vi "WLAN - niVST - RFSG - Create and Down Load Wfm.vi"(0 "instrument handle":refnum<k15>, 1 "Waveform Generation Settings":T2[](array[typedef])=[{"Standard"=0, "Channel Bandwidth (Hz)"=20000000.0, "Idle Interval (s)"=0.0001, "MCS Index"=0, "80211n PLCP Frame Format"=0, "Payload Data Length (bytes)"=100, "OFDM Data Rate (Mbps)"=0, "DSSS Data Rate (Mbps)"=0, "Wfm_Index"=0}, {"Standard"=0, "Channel Bandwidth (Hz)"=20000000.0, "Idle Interval (s)"=0.001, "MCS Index"=0, "80211n PLCP Frame Format"=0, "Payload Data Length (bytes)"=200, "OFDM Data Rate (Mbps)"=2, "DSSS Data Rate (Mbps)"=0, "Wfm_Index"=1}, {"Standard"=0, "Channel Bandwidth (Hz)"=20000000.0, "Idle Interval (s)"=0.0001, "MCS Index"=0, "80211n PLCP Frame Format"=0, "Payload Data Length (bytes)"=300, "OFDM Data Rate (Mbps)"=4, "DSSS Data Rate (Mbps)"=0, "Wfm_Index"=2}, {"Standard"=0, "Channel Bandwidth (Hz)"=20000000.0, "Idle Interval (s)"=0.0001, "MCS Index"=0, "80211n PLCP Frame Format"=0, "Payload Data Length (bytes)"=600, "OFDM Data Rate (Mbps)"=7, "DSSS Data Rate (Mbps)"=0, "Wfm_Index"=3}, {"Standard"=1, "Channel Bandwidth (Hz)"=20000000.0, "Idle Interval (s)"=0.0001, "MCS Index"=0, "80211n PLCP Frame Format"=0, "Payload Data Length (bytes)"=50, "OFDM Data Rate (Mbps)"=0, "DSSS Data Rate (Mbps)"=0, "Wfm_Index"=4}, {"Standard"=1, "Channel Bandwidth (Hz)"=20000000.0, "Idle Interval (s)"=0.0001, "MCS Index"=0, "80211n PLCP Frame Format"=0, "Payload Data Length (bytes)"=200, "OFDM Data Rate (Mbps)"=0, "DSSS Data Rate (Mbps)"=4, "Wfm_Index"=5}, {"Standard"=3, "Channel Bandwidth (Hz)"=20000000.0, "Idle Interval (s)"=0.0001, "MCS Index"=0, "80211n PLCP Frame Format"=0, "Payload Data Length (bytes)"=80, "OFDM Data Rate (Mbps)"=0, "DSSS Data Rate (Mbps)"=0, "Wfm_Index"=6}, {"Standard"=3, "Channel Bandwidth (Hz)"=20000000.0, "Idle Interval (s)"=0.0001, "MCS Index"=4, "80211n PLCP Frame Format"=0, "Payload Data Length (bytes)"=200, "OFDM Data Rate (Mbps)"=0, "DSSS Data Rate (Mbps)"=0, "Wfm_Index"=7}, {"Standard"=3, "Channel Bandwidth (Hz)"=20000000.0, "Idle Interval (s)"=0.0001, "MCS Index"=7, "80211n PLCP Frame Format"=0, "Payload Data Length (bytes)"=700, "OFDM Data Rate (Mbps)"=0, "DSSS Data Rate (Mbps)"=0, "Wfm_Index"=8}, {"Standard"=0, "Channel Bandwidth (Hz)"=20000000.0, "Idle Interval (s)"=0.0001, "MCS Index"=0, "80211n PLCP Frame Format"=0, "Payload Data Length (bytes)"=60, "OFDM Data Rate (Mbps)"=0, "DSSS Data Rate (Mbps)"=0, "Wfm_Index"=9}, {"Standard"=0, "Channel Bandwidth (Hz)"=20000000.0, "Idle Interval (s)"=0.0001, "MCS Index"=0, "80211n PLCP Frame Format"=0, "Payload Data Length (bytes)"=200, "OFDM Data Rate (Mbps)"=2, "DSSS Data Rate (Mbps)"=0, "Wfm_Index"=10}, {"Standard"=0, "Channel Bandwidth (Hz)"=20000000.0, "Idle Interval (s)"=0.0001, "MCS Index"=0, "80211n PLCP Frame Format"=0, "Payload Data Length (bytes)"=300, "OFDM Data Rate (Mbps)"=4, "DSSS Data Rate (Mbps)"=0, "Wfm_Index"=11}, {"Standard"=0, "Channel Bandwidth (Hz)"=20000000.0, "Idle Interval (s)"=0.0001, "MCS Index"=0, "80211n PLCP Frame Format"=0, "Payload Data Length (bytes)"=600, "OFDM Data Rate (Mbps)"=7, "DSSS Data Rate (Mbps)"=0, "Wfm_Index"=12}, {"Standard"=3, "Channel Bandwidth (Hz)"=20000000.0, "Idle Interval (s)"=0.0001, "MCS Index"=0, "80211n PLCP Frame Format"=0, "Payload Data Length (bytes)"=80, "OFDM Data Rate (Mbps)"=0, "DSSS Data Rate (Mbps)"=0, "Wfm_Index"=13}, {"Standard"=3, "Channel Bandwidth (Hz)"=20000000.0, "Idle Interval (s)"=0.0001, "MCS Index"=4, "80211n PLCP Frame Format"=0, "Payload Data Length (bytes)"=300, "OFDM Data Rate (Mbps)"=0, "DSSS Data Rate (Mbps)"=0, "Wfm_Index"=14}, {"Standard"=3, "Channel Bandwidth (Hz)"=20000000.0, "Idle Interval (s)"=0.0001, "MCS Index"=7, "80211n PLCP Frame Format"=0, "Payload Data Length (bytes)"=600, "OFDM Data Rate (Mbps)"=0, "DSSS Data Rate (Mbps)"=0, "Wfm_Index"=15}, {"Standard"=3, "Channel Bandwidth (Hz)"=40000000.0, "Idle Interval (s)"=0.0001, "MCS Index"=0, "80211n PLCP Frame Format"=0, "Payload Data Length (bytes)"=120, "OFDM Data Rate (Mbps)"=0, "DSSS Data Rate (Mbps)"=0, "Wfm_Index"=16}, {"Standard"=3, "Channel Bandwidth (Hz)"=40000000.0, "Idle Interval (s)"=0.0001, "MCS Index"=4, "80211n PLCP Frame Format"=0, "Payload Data Length (bytes)"=400, "OFDM Data Rate (Mbps)"=0, "DSSS Data Rate (Mbps)"=0, "Wfm_Index"=17}, {"Standard"=3, "Channel Bandwidth (Hz)"=40000000.0, "Idle Interval (s)"=0.0001, "MCS Index"=7, "80211n PLCP Frame Format"=0, "Payload Data Length (bytes)"=1024, "OFDM Data Rate (Mbps)"=0, "DSSS Data Rate (Mbps)"=0, "Wfm_Index"=18}] {"DSSS Data Rate (Mbps)" items=["1", "2", "5.5 CCK", "5.5 PBCC", "11 CCK", "11 PBCC", "22", "33"]; "OFDM Data Rate (Mbps)" items=["6", "9", "12", "18", "24", "36", "48", "54"]; "80211n PLCP Frame Format" items=["Mixed Format", "Greenfield Format"]; "Standard" items=["80211A/G/J/P OFDM", "80211B/G DSSS", "80211G DSSSOFDM", "80211N MIMOOFDM", "80211AC MIMOOFDM"]}, 2 "ScriptName<index>":string="WLANRxTesting", 11 "error in":errorcluster, 12 "Address String":string="00:90:4C:C5:12:38", 13 "numPackets":i32=100) -> (4 "instrument handle":refnum<k15>, 6 "Test Paramaters":T1[](array[typedef]) {"OFDM Data Rate (Mbps)" items=["6", "9", "12", "18", "24", "36", "48", "54"]; "DSSS Data Rate (Mbps)" items=["1", "2", "5.5 CCK", "5.5 PBCC", "11 CCK", "11 PBCC", "22", "33"]; "80211n PLCP Frame Format" items=["Mixed Format", "Greenfield Format"]}, 15 "error out":errorcluster)   [LabVIEW 2011]
uses:
  TV/RW/Includes/WLAN - TV - RW - INC - Rx_PER_Wfm_Settings.ctl
  TV/RW/Includes/WLAN - TV - RW - INC - RxTestParameters.ctl
  <instrlib>/niRFSG/niRFSG.llb/niRFSG Write Arb Waveform (Complex Input).vi
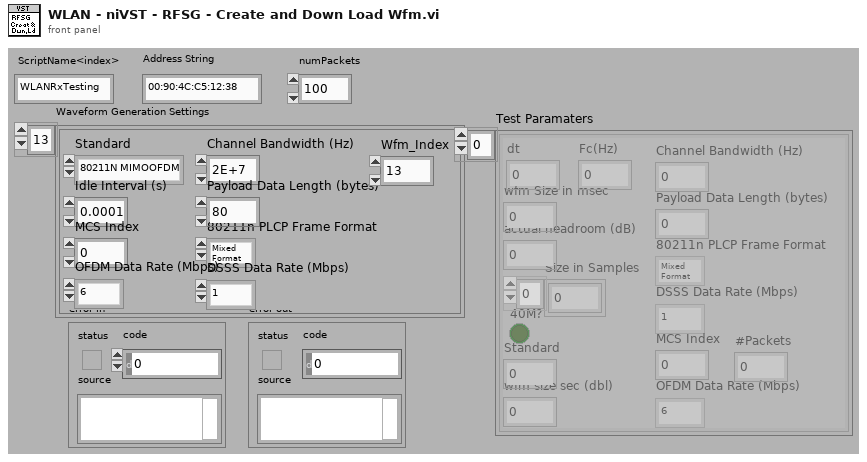
[diagram p1: front panel]
types:
  T1 = typedef "WLAN - TV - RW - INC - RxTestParameters.ctl" = cluster{"wfm Size in msec":i32, "actual headroom (dB)":dbl, "Size in Samples":i32[], "40M?":bool, "Standard ":i32, "wfm size sec (dbl)":dbl, "dt":dbl, "Channel Bandwidth (Hz)":dbl, "Payload Data Length (bytes)":i32, "80211n PLCP Frame Format":i32, "DSSS Data Rate (Mbps)":i32, "OFDM Data Rate (Mbps)":i32, "MCS Index":i32, "Fc(Hz)":dbl, "#Packets":i32}
  T2 = typedef "WLAN - TV - RW - INC - Rx_PER_Wfm_Settings.ctl" = cluster{"Standard":i32, "Channel Bandwidth (Hz)":dbl, "Idle Interval (s)":dbl, "MCS Index":i32, "80211n PLCP Frame Format":i32, "Payload Data Length (bytes)":i32, "OFDM Data Rate (Mbps)":i32, "DSSS Data Rate (Mbps)":i32, "Wfm_Index":i32}
  T3 = cluster{"Waveforms":cluster{"t0":dbl, "dt":dbl, "Y":cdb[]}[], "wfm Size in msec":i32, "actual headroom (dB)":dbl, "Size in Samples":i32[], "40M?":bool, "Standard ":i32, "wfm size sec (dbl)":dbl}[]
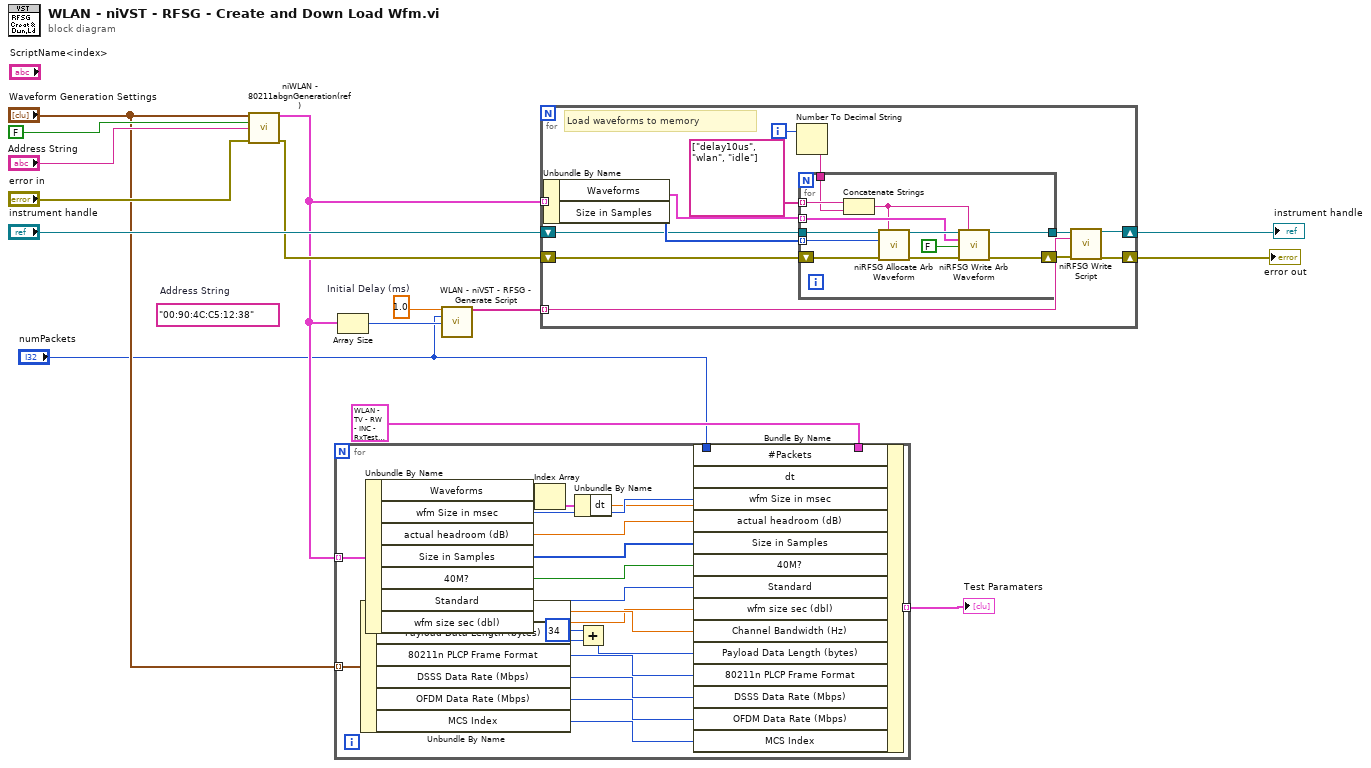
[diagram p0: block diagram]
diagram:
  (unwired) "00:90:4C:C5:12:38"  # Address String
  w15 = 1.0  # Initial Delay (ms)
  n1 = call "niWLAN - 80211abgnGeneration(ref).vi"("Waveform Generation Settings"="Waveform Generation Settings", "Without ACK ?"=FALSE ("w/ ACK"), "Address String"="Address String", "error in"="error in") -> ("Output"=w7:T3, "error out"=w8:errorcluster)  [unwired: 10 in]
  n2 = for {
    tunnel: w7 -> [w36] mode=indexing
    tunnel: T1 {"wfm Size in msec"=0, "actual headroom (dB)"=0.0, "Size in Samples"=[], "40M?"=FALSE, "Standard "=0, "wfm size sec (dbl)"=0.0, "dt"=0.0, "Channel Bandwidth (Hz)"=0.0, "Payload Data Length (bytes)"=0, "80211n PLCP Frame Format"=0, "DSSS Data Rate (Mbps)"=0, "OFDM Data Rate (Mbps)"=0, "MCS Index"=0, "Fc(Hz)"=0.0, "#Packets"=0} ("Cluster") -> [w37]
    tunnel: [w28] -> w4 mode=indexing
    tunnel: "Waveform Generation Settings" -> [w27] mode=indexing
    tunnel: "numPackets" -> [w18]
    n3 = Unbundle By Name(w27) -> ("Channel Bandwidth (Hz)"=w26:dbl, "Payload Data Length (bytes)"=w25:i32, "80211n PLCP Frame Format"=w24:i32, "DSSS Data Rate (Mbps)"=w23:i32, "OFDM Data Rate (Mbps)"=w22:i32, "MCS Index"=w21:i32)
    n4 = Unbundle By Name(w36) -> ("Waveforms"=w35:cluster{"t0":dbl, "dt":dbl, "Y":cdb[]}[], "wfm Size in msec"=w33:i32, "actual headroom (dB)"=w29:dbl, "Size in Samples"=w30:i32[], "40M?"=w31:bool, "Standard"=w32:i32, "wfm size sec (dbl)"=w16:dbl)
    n5 = Index Array(array=w35) -> (element=w34:cluster{"t0":dbl, "dt":dbl, "Y":cdb[]})  [unwired: 1 in]
    n6 = Unbundle By Name(w34) -> ("dt"=w17:dbl)
    n7 = Add(x=34, y=w25) -> (x+y=w20:i32)
    n8 = Bundle By Name(cluster=w37, "#Packets"=w18, "dt"=w17, "wfm Size in msec"=w33, "actual headroom (dB)"=w29, "Size in Samples"=w30, "40M?"=w31, "Standard"=w32, "wfm size sec (dbl)"=w16, "Channel Bandwidth (Hz)"=w26, "Payload Data Length (bytes)"=w20, "80211n PLCP Frame Format"=w24, "DSSS Data Rate (Mbps)"=w23, "OFDM Data Rate (Mbps)"=w22, "MCS Index"=w21) -> (w28:T1)
  }
  "Test Paramaters" <- w4
  n9 = Array Size(array=w7) -> (size(s)=w13:i32)
  n10 = call "WLAN - niVST - RFSG - Generate Script.vi"("Initial Delay (ms)"=w15, "Number of Packets"="numPackets", "Number of Scripts"=w13) -> ("Array"=w14:string[])  [unwired: 12 in]
  n11 = for {
    tunnel: w7 -> [w49] mode=indexing
    shift-right: [w41] -> w1
    shift-left: "instrument handle" -> [w39]
    shift-right: [w40] -> w2
    shift-left: w8 -> [w38]
    tunnel: w14 -> [w44] mode=indexing
    i -> [w46]
    # "Load waveforms to memory"
    n12 = Unbundle By Name(w49) -> ("Waveforms"=w47:cluster{"t0":dbl, "dt":dbl, "Y":cdb[]}[], "Size in Samples"=w48:i32[])
    n13 = Number To Decimal String(number=w46) -> (decimal integer string=w45:string)  [unwired: 1 in]
    n14 = for {
      tunnel: [w59] -> w43
      tunnel: w39 -> [w56]
      shift-right: [w58] -> w42
      shift-left: w38 -> [w57]
      tunnel: string[] ["delay10us", "wlan", "idle"] -> [w53] mode=indexing
      tunnel: w48 -> [w55] mode=indexing
      tunnel: w47 -> [w54] mode=indexing
      tunnel: w45 -> [w52]
      n15 = Concatenate Strings(w53, w52) -> (w51:string)
      n16 = call <instrlib>:"niRFSG Allocate Arb Waveform.vi"("instrument handle"=w56, "name"=w51, "size in samples"=w55, "error in"=w57) -> ("instrument handle out"=w61:refnum<k15>, "error out"=w60:errorcluster)  [unwired: 10 in]
      n17 = call-poly <instrlib>:"niRFSG Write Arb Waveform.vi"("instrument handle"=w61, "name"=w51, "IQ waveform"=w54, "use waveform dt for IQ rate?"=FALSE, "error in"=w60) -> ("instrument handle out"=w59:refnum<k15>, "error out"=w58:errorcluster)  [unwired: 9 in]
    }
    n18 = call <instrlib>:"niRFSG Write Script.vi"("instrument handle"=w43, "script"=w44, "error in"=w42) -> ("instrument handle out"=w41:refnum<k15>, "error out"=w40:errorcluster)  [unwired: 11 in]
  }
  "error out" <- w2
  "instrument handle" <- w1
